vi "NI OCR-Training Window.vi"(8 "error in":errorcluster, 11 "Image In":T1) -> (0 "error out":errorcluster, 1 "OK?":bool, 2 "Character Out":string, 3 "Image Out":T1)   [LabVIEW 2016]
uses:
  <vilib>/vision/Image Controls.llb/IMAQ Image.ctl
  <vilib>/Utility/miscctls.llb/LVPointTypeDef.ctl
panel:
  in  "Cancel":bool
  in  "Ok":bool
  in  "Character":string
  out "Display Image":T1(plugin-control)
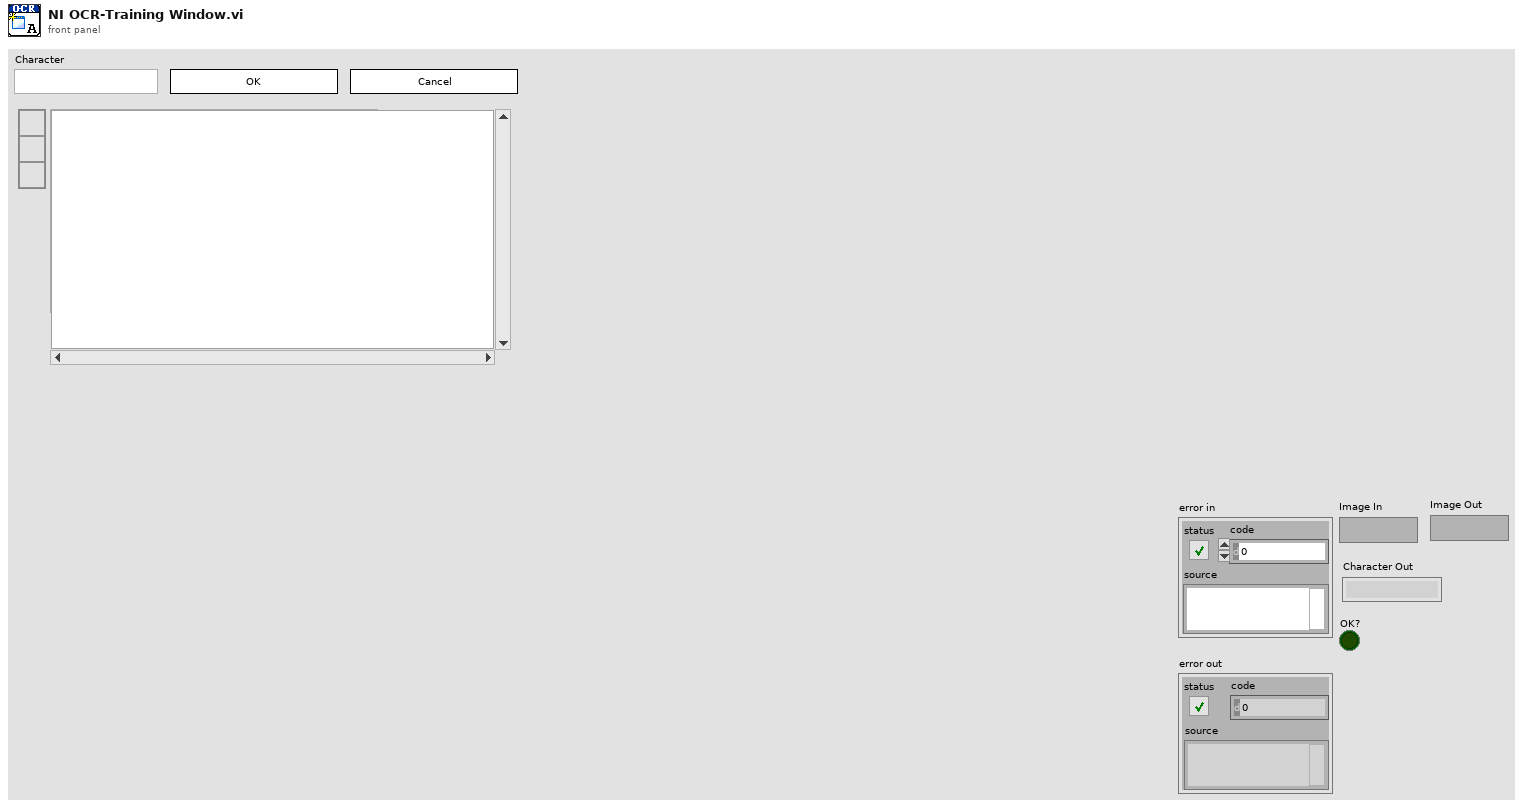
[diagram p1: front panel]
types:
  T1 = typedef "IMAQ Image.ctl" = refnum<image>
  T2 = typedef "LVPointTypeDef.ctl" = cluster{"Horizontal":i16, "Vertical":i16}
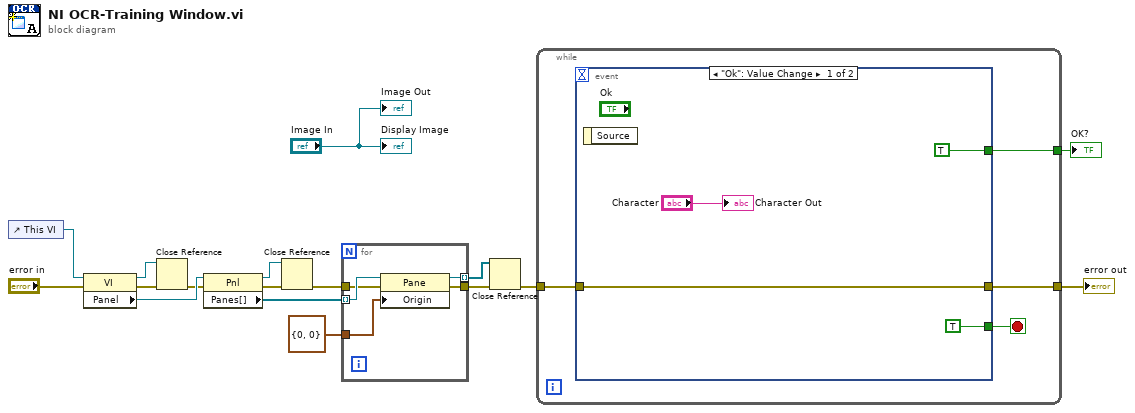
[diagram p0: block diagram]
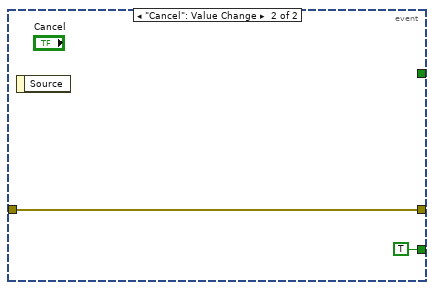
[diagram p2: hidden frame]
diagram:
  n1 = control-ref of="This VI"() -> (w9:refnum<vi>)
  n2 = property class="VI"(reference=w9, error in="error in") -> (reference out=w6:refnum<vi>, error out=w7:errorcluster, "Panel"=w17:refnum<vi>)
  n3 = Close Reference(reference=w6, error in (no error)=w7) -> (error out=w5:errorcluster)
  n4 = property class="Pnl"(reference=w17, error in=w5) -> (reference out=w13:refnum<vi>, error out=w14:errorcluster, "Panes[]"=w16:refnum<vi>[])
  n5 = Close Reference(reference=w13, error in (no error)=w14) -> (error out=w12:errorcluster)
  n6 = for {
    tunnel: w12 -> [w21]
    tunnel: w16 -> [w22] mode=indexing
    tunnel: T2 {"Horizontal"=0, "Vertical"=0} ("Origin") -> [w20]
    tunnel: [w19] -> w11
    tunnel: [w18] -> w10 mode=indexing
    n7 = property class="Pane"(reference=w22, error in=w21, "Origin"=w20) -> (reference out=w18:refnum<vi>, error out=w19:errorcluster)
  }
  n8 = Close Reference(reference=w10, error in (no error)=w11) -> (error out=w4:errorcluster)
  n9 = while {
    tunnel: w4 -> [w26]
    tunnel: [w25] -> w2
    tunnel: [w23] -> w3
    stop <- w24 stop-if-true
    n10 = event shown="[0] \"Ok\": Value Change" {
      selector: _ -> [_ _]
      dyn-events: _ -> [_ _]
      timeout: _ -> [_ _]
      tunnel: w26 -> [w29 w32]
      tunnel: [w29 w32] -> w25
      tunnel: [TRUE TRUE] -> w24
      tunnel: [TRUE _] -> w23
      event "Ok": Value Change {
        n11 = event-data() -> ()  [unwired: 1 in, 1 out]
        "Character Out" <- "Character"
      }
      event "Cancel": Value Change {
        n12 = event-data() -> ()  [unwired: 1 in, 1 out]
      }
    }
  }
  "error out" <- w2
  "OK?" <- w3
  "Display Image" <- "Image In"
  "Image Out" <- "Image In"
